vi "Model--Reorder.vi"(8 "error in":errorcluster, 11 "Selector in":refnum<class "Selector.lvclass">) -> (0 "error out":errorcluster, 3 "Selector out":refnum<class "Selector.lvclass">)   [LabVIEW 2019, in "Selector.lvclass"]
uses:
  Selector.lvclass
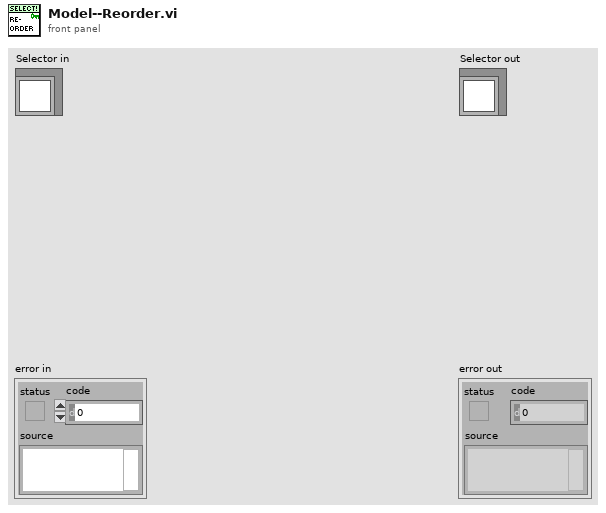
[diagram p1: front panel]
types:
  T1 = typedef "Selector.lvclass/Item.ctl" = cluster{"Name":string, "Group":string, "Enabled":bool}
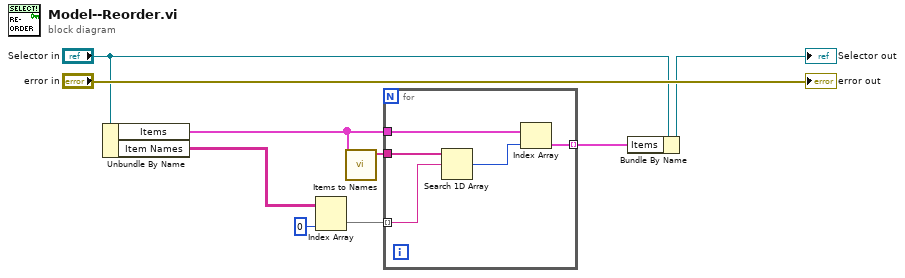
[diagram p0: block diagram]
diagram:
  n1 = Unbundle By Name("Selector in") -> ("Items"=w4:T1[], "Item Names"=w1:string[][])
  n2 = Index Array(array=w1, index (col)=0 ("disabled index (col)")) -> (element=w6:string[])  [unwired: 1 in]
  n3 = call "Items to Names.vi"("Items"=w4) -> ("Names"=w8:string[])  [unwired: 6 in]
  n4 = for {
    tunnel: w4 -> [w12]
    tunnel: w8 -> [w14]
    tunnel: w6 -> [w13] mode=indexing
    tunnel: [w10] -> w5 mode=indexing
    n5 = Search 1D Array(1D array=w14, element=w13) -> (index of element=w11:i32)  [unwired: 1 in]
    n6 = Index Array(array=w12, index=w11) -> (element=w10:T1)
  }
  n7 = Bundle By Name(cluster="Selector in", "Items"=w5) -> (→"Selector out":refnum<class "Selector.lvclass">)
  "error out" <- "error in"
